vi "Release-status-notifs.vi"(8 "error in (no error)":errorcluster, 11 "Object ref in":T1) -> (0 "error out":errorcluster, 3 "Object ref out":T1)   [LabVIEW 2013, in "SLMControl.lvlib" / "SC-Main.lvclass"]
uses:
  SC-Main.lvclass
  Object-reference.ctl
  SC-Main.lvclass/SC-Main.ctl
  Read Abort.vi
  Read Exit.vi
  Read Deposition notif.vi
  Read Lasing notif.vi
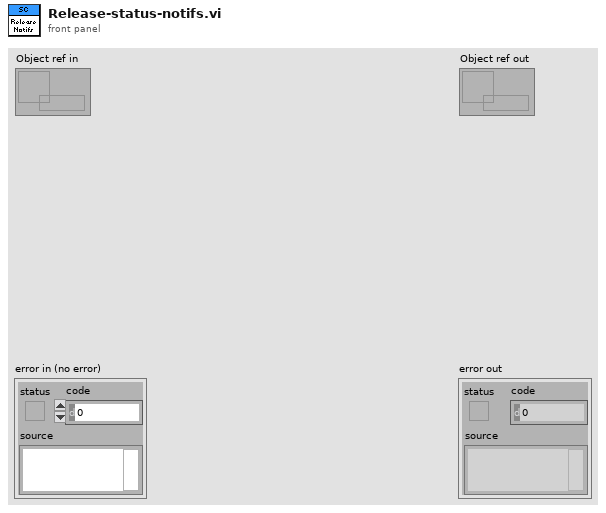
[diagram p1: front panel]
types:
  T1 = typedef "SLMControl.lvlib/SC-Main.lvclass/Object-reference.ctl" = refnum<data-value>
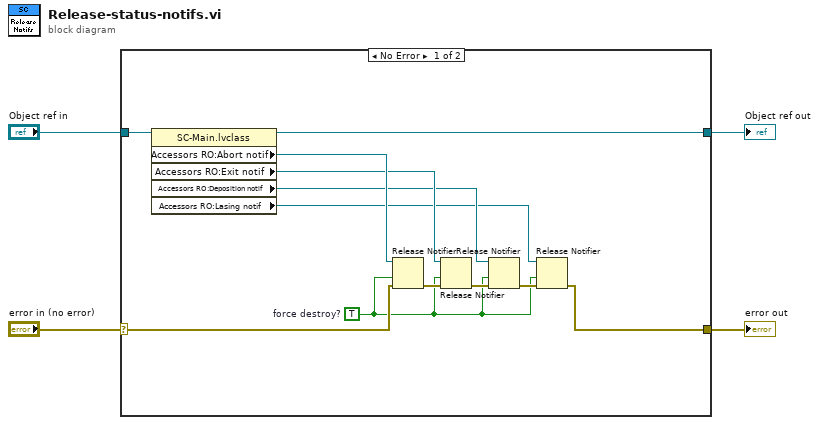
[diagram p0: block diagram]
diagram:
  n1 = case shown="No Error" "error in (no error)" {
    selector: "error in (no error)" -> [w13 w18]
    tunnel: [w8 w18] -> w3
    tunnel: [w15 w17] -> w1
    tunnel: "Object ref in" -> [w16 w17]
    frame No Error {
      w7 = TRUE  # force destroy?
      n2 = property class="SC-Main.lvclass"(reference=w16) -> (reference out=w15:T1, "Accessors RO:Abort notif"=w14:refnum<notifier>, "Accessors RO:Exit notif"=w11:refnum<notifier>, "Accessors RO:Deposition notif"=w6:refnum<notifier>, "Accessors RO:Lasing notif"=w5:refnum<notifier>)  [unwired: 1 in, 1 out]
      n3 = Release Notifier(notifier=w14, force destroy? (F)=w7, error in (no error)=w13) -> (error out=w12:errorcluster)  [unwired: 2 out]
      n4 = Release Notifier(notifier=w11, force destroy? (F)=w7, error in (no error)=w12) -> (error out=w10:errorcluster)  [unwired: 2 out]
      n5 = Release Notifier(notifier=w6, force destroy? (F)=w7, error in (no error)=w10) -> (error out=w9:errorcluster)  [unwired: 2 out]
      n6 = Release Notifier(notifier=w5, force destroy? (F)=w7, error in (no error)=w9) -> (error out=w8:errorcluster)  [unwired: 2 out]
    }
    frame Error {
    }
  }
  "error out" <- w3
  "Object ref out" <- w1
